vi "UART FGV Loop.vi"() -> ()   [LabVIEW 2017]
uses:
  <vilib>/myRIO/Instrument Drivers/Onboard IO/UART/typedef/VISA Configuration.ctl
  <vilib>/myRIO/Instrument Drivers/Onboard IO/DIO/typedefs/DIO Reference.ctl
  <vilib>/myRIO/Common/Instrument Driver Framework/Utilities/typedefs/myRIO Generic Hardware Reference.ctl
  <vilib>/myRIO/Common/Instrument Driver Framework/Utilities/typedefs/Hardware Version Enum.ctl
  <vilib>/myRIO/Common/Instrument Driver Framework/Utilities/typedefs/myRIO v1.0 Reference.ctl
  <vilib>/myRIO/Common/Instrument Driver Framework/Utilities/typedefs/Generic FPGA Reference.ctl
  <vilib>/myRIO/Common/Instrument Driver Framework/myRIO v1.0/DIO/typedefs/DIO Channels List.ctl
  <vilib>/myRIO/Common/Instrument Driver Framework/myRIO v1.0/DIO/typedefs/DIO Channels Enum.ctl
  <vilib>/userdefined/High Color/nirio_resource_hc.ctl
  <vilib>/myRIO/Common/Instrument Driver Framework/Utilities/vis/Is FPGA Ref Available.vi
  <vilib>/myRIO/Common/Instrument Driver Framework/myRIO v1.0/DIO/vis/myRIO v1.1 Open DIO.vi
  <vilib>/myRIO/Instrument Drivers/Onboard IO/DIO/vis/Write.vi
  <vilib>/myRIO/Common/Instrument Driver Framework/Utilities/vis/Validate Channels.vi
  <vilib>/myRIO/Common/Instrument Driver Framework/myRIO v1.0/DIO/vis/myRIO v1.0 Reserve DIO.vi
  <vilib>/Analysis/baseanly.llb/Outer Product.vi
  <vilib>/Analysis/baseanly.llb/Real Outer Product.vi
  <vilib>/robotics/Kinematics/Create Lie Group Matrix.vi
  <vilib>/myRIO/Common/Instrument Driver Framework/myRIO v1.0/Resource Manager/vis/myRIO v1.0 Reserve Channel List.vi
  <vilib>/myRIO/Common/Instrument Driver Framework/myRIO v1.0/DIO/vis/myRIO v1.0 Build MUX Configuration DIO.vi
  <vilib>/myRIO/Common/Instrument Driver Framework/myRIO v1.0/Resource Manager/vis/myRIO v1.0 Reserve Channel.vi
  <vilib>/myRIO/Common/Instrument Driver Framework/myRIO v1.0/Resource Manager/vis/myRIO v1.0 Unreserve Channel.vi
  <vilib>/myRIO/Common/Instrument Driver Framework/myRIO v1.0/Resource Manager/vis/myRIO v1.0 Create Configuration List.vi
  <vilib>/myRIO/Common/Instrument Driver Framework/myRIO v1.0/Resource Manager/vis/myRIO v1.0 Build Mutex Name.vi
  <vilib>/Utility/VariantDataType/GetNumericInfo.vi
  <vilib>/Utility/error.llb/Error Cluster From Error Code.vi
  <vilib>/myRIO/Common/Instrument Driver Framework/myRIO v1.0/myRIO v1.1 Open.vi
  <vilib>/myRIO/Common/Instrument Driver Framework/Utilities/vis/IO Manager.vi
  <vilib>/myRIO/Common/Instrument Driver Framework/Utilities/vis/Configuration Manager.vi
  <vilib>/myRIO/Common/Instrument Driver Framework/myRIO v1.0/Resource Manager/vis/myRIO v1.0 Configure IO.vi
  <vilib>/myRIO/Common/Instrument Driver Framework/myRIO v1.0/myRIO v1.0 Close.vi
  <vilib>/myRIO/Common/Instrument Driver Framework/myRIO v1.0/DIO/vis/myRIO v1.0 Write DIO.vi
  <vilib>/Analysis/Matrix/Numeric/Multiply/Multiply.vi
  <vilib>/Analysis/Matrix/Numeric/Multiply/Multiply - RM,R.vi
  <vilib>/Analysis/Matrix/Numeric/Multiply/Multiply - R,RM.vi
  <vilib>/Analysis/Matrix/Numeric/Add/Add.vi
  <vilib>/Analysis/Matrix/Numeric/Add/Add - RM,RM.vi
  <vilib>/myRIO/Express VI/Onboard IO/DO/DO Express VI.xnode
  <vilib>/myRIO/Instrument Drivers/Onboard IO/DIO/vis/myRIO DIO Open.xnode
  <vilib>/myRIO/Instrument Drivers/Onboard IO/DIO/DIO.lvlib
  <vilib>/NI/Tools/String/Tools_String.lvlib
  <vilib>/robotics/Kinematics/NI_Kinematics.lvlib
  <vilib>/myRIO/Instrument Drivers/Onboard IO/UART/UART.lvlib
panel:
  out "Waveform Chart":cluster{"roll":dbl, "pitch":dbl, "yaw":dbl}[](graph)
  out "token array":string[](array[string])
  in  "reset time (ms)":u32=300
  in  "boot time (ms)":u32=1200
  out "error?":bool
  in  "stop":bool
  out "read buffer":string
  in  "Read mode":enum16{"Read all", "Get latest value"}(ring)=enum."Get latest value"
  in  "VISA resource name in":refnum<visa-resource-name>="ASRL2::INSTR"
  out "timeout (10sec)":u32
  in  "input cluster":T1={"baud rate (9600)"=115200, "data bits (8)"=8, "parity (0:none)"=enum."None", "stop bits (10: 1 bit)"=10, "flow control (0:none)"=0, "termination char\n(0xA = '\\n' = LF) "=10, "Enable Termination\nChar (T)"=TRUE, "timeout (10sec)"=1000} {"termination char\n(0xA = '\\n' = LF)" format="%.0x"; "flow control (0:none)" items=["None", "XON/XOFF", "RTS/CTS", "XON/XOFF & RTS/CTS", "DTR/DSR", "XON/XOFF & DTR/DSR"]; "stop bits (10: 1 bit)" items=["1.0"=10, "1.5"=15, "2.0"=20]; "data bits (8)" min=5 max=8 step=1}
  out "error out":errorcluster
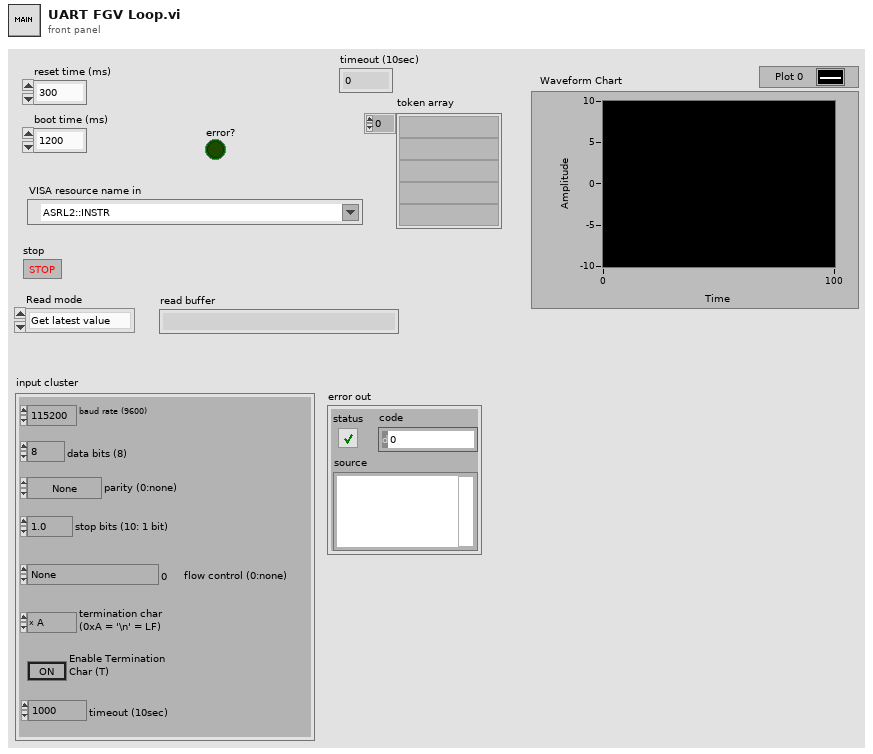
[diagram p1: front panel]
types:
  T1 = typedef "UART.lvlib/VISA Configuration.ctl" = cluster{"baud rate (9600)":u32, "data bits (8)":u16, "parity (0:none)":enum16{"None", "Odd", "Even", "Mark", "Space"}, "stop bits (10: 1 bit)":u16, "flow control (0:none)":u16, "termination char\n(0xA = '\\n' = LF) ":u8, "Enable Termination\nChar (T)":bool, "timeout (10sec)":u32}
  T2 = typedef "DIO.lvlib/DIO Reference.ctl" = cluster{"myRIO Reference":T3, "DIO Channels List":T7}
  T3 = typedef "myRIO Generic Hardware Reference.ctl" = cluster{"myRIO Model":T4, "myRIO Hardware Reference":T5}
  T4 = typedef "Hardware Version Enum.ctl" = enum16{"Unknown", "myRIO-1900", "myRIO-1950", "roboRIO", "NI ELVIS RIO CM"}
  T5 = typedef "myRIO v1.0 Reference.ctl" = cluster{"Generic FPGA Reference":T6, "Allow multiple opens":bool}
  T6 = typedef "Generic FPGA Reference.ctl" = refnum<k20>
  T7 = typedef "DIO Channels List.ctl" = T8[]
  T8 = typedef "DIO Channels Enum.ctl" = enum16{"Not Connected", "C/DIO0", "C/DIO1", "C/DIO2", "C/DIO3", "C/DIO4", "C/DIO5", "C/DIO6", "C/DIO7", "A/DIO0", "A/DIO1", "A/DIO2", "A/DIO3", "A/DIO4", "A/DIO5", "A/DIO6", "A/DIO7", "A/DIO8", "A/DIO9", "A/DIO10", "A/DIO11", "A/DIO12", "A/DIO13", "A/DIO14", "A/DIO15", "B/DIO0", "B/DIO1", "B/DIO2", "B/DIO3", "B/DIO4", "B/DIO5", "B/DIO6", "B/DIO7", "B/DIO8", "B/DIO9", "B/DIO10", "B/DIO11", "B/DIO12", "B/DIO13", "B/DIO14", "B/DIO15", "LED0", "LED1", "LED2", "LED3", "Button0", "DIO/DIO0", "DIO/DIO1", "DIO/DIO2", "DIO/DIO3", "DIO/DIO4", "DIO/DIO5", "DIO/DIO6", "DIO/DIO7", "DIO/DIO8", "DIO/DIO9", "SPI/CS0", "SPI/CS1", "SPI/CS2", "SPI/CS3", "LED RADIO (Green)", "LED RADIO (Red)", "LED COMM (Green)", "LED COMM (Red)", "LED MODE (Green)", "LED MODE (Red)"}
  T9 = typedef "nirio_resource_hc.ctl" = tag
  T10 = typedef "NI_Matrix.lvlib/RealMatrix.ctl" = dbl[][]
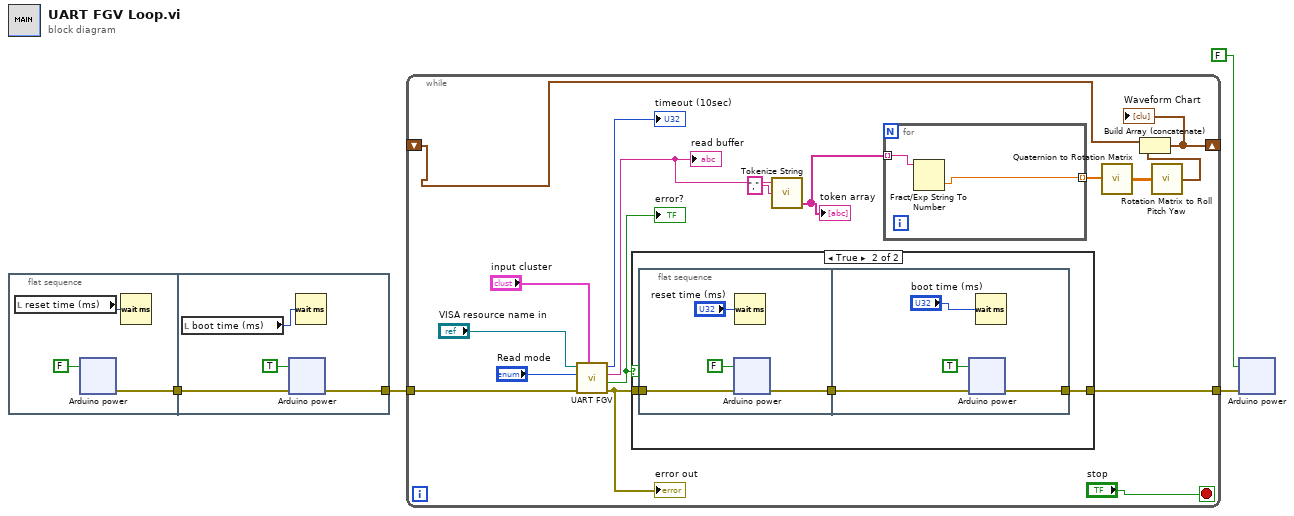
[diagram p0: block diagram]
diagram:
  n1 = flat-sequence {
    tunnel: [w6] -> w4
    tunnel: w4 -> [w45]
    tunnel: [w44] -> w3
    frame #0 {
      n2 = local read "reset time (ms)"() -> (w5:u32)
      n3 = xnode "Arduino power"("B/DIO0 (Pin 11)"=FALSE) -> ("error out"=w6:errorcluster)  [unwired: 1 in]
      n4 = Wait (ms)(milliseconds to wait=w5) -> ()  [unwired: 1 out]
    }
    frame #1 {
      n5 = local read "boot time (ms)"() -> (w43:u32)
      n6 = xnode "Arduino power"("error in (no error)"=w45, "B/DIO0 (Pin 11)"=TRUE) -> ("error out"=w44:errorcluster)
      n7 = Wait (ms)(milliseconds to wait=w43) -> ()  [unwired: 1 out]
    }
  }
  n8 = while {
    tunnel: w3 -> [w92]
    tunnel: [w91] -> w2
    shift-right: [w82] -> _
    shift-left: _ -> [w83]
    stop <- "stop" stop-if-true
    n9 = call "UART FGV.vi"("input cluster"="input cluster", "error in (no error)"=w92, "Read mode"="Read mode", "VISA Refnum in"="VISA resource name in") -> ("error out"=w90:errorcluster, "error? out"=w93:bool, "read buffer"=w89:string, "timeout (10sec)"=→"timeout (10sec)":u32)  [unwired: 4 in]
    "error out" <- w90
    "read buffer" <- w89
    "error?" <- w93
    n10 = case shown="True" w93 {
      tunnel: [w101 w103] -> w91
      tunnel: w90 -> [w101 w102]
      frame False {
      }
      frame True {
        n11 = flat-sequence {
          tunnel: [w107] -> w104
          tunnel: w102 -> [w106]
          tunnel: w104 -> [w146]
          tunnel: [w145] -> w103
          frame #0 {
            n12 = xnode "Arduino power"("error in (no error)"=w106, "B/DIO0 (Pin 11)"=FALSE) -> ("error out"=w107:errorcluster)
            n13 = Wait (ms)(milliseconds to wait="reset time (ms)") -> ()  [unwired: 1 out]
          }
          frame #1 {
            n14 = xnode "Arduino power"("error in (no error)"=w146, "B/DIO0 (Pin 11)"=TRUE) -> ("error out"=w145:errorcluster)
            n15 = Wait (ms)(milliseconds to wait="boot time (ms)") -> ()  [unwired: 1 out]
          }
        }
      }
    }
    n16 = call <vilib>:"Tokenize String.vi"("delimiter ([\\s\\t\\n\\r]+)"="," ("delimiter ([\\s\\t\\n\\r]+)"), "input string"=w89) -> ("token array"=w87:string[])  [unwired: 2 in, 1 out]
    "token array" <- w87
    n17 = for {
      tunnel: w87 -> [w100] mode=indexing
      tunnel: [w99] -> w86 mode=indexing
      n18 = Fract/Exp String To Number(string=w100) -> (number=w99:dbl)  [unwired: 3 in, 1 out]
    }
    n19 = call <vilib>:"Quaternion to Rotation Matrix.vi"("quaternion"=w86) -> ("rotation matrix"=w85:T10)
    n20 = call <vilib>:"Rotation Matrix to Roll Pitch Yaw.vi"("rotation matrix"=w85) -> ("angles"=w84:cluster{"roll":dbl, "pitch":dbl, "yaw":dbl})
    n21 = Build Array (concatenate)(w83, w84) -> (w82:cluster{"roll":dbl, "pitch":dbl, "yaw":dbl}[])
    "Waveform Chart" <- w82
  }
  n22 = xnode "Arduino power"("error in (no error)"=w2, "B/DIO0 (Pin 11)"=FALSE) -> ()  [unwired: 1 out]
